vi "EMC_REL_Move.vi"(8 "error in (no error)":errorcluster, 10 "Motion Parameters":T1={"position"=1000.0, "velocity"=1000.0, "acceleration"=10000.0, "deceleration"=10000.0, "accel. jerk"=10000.0, "decel. jerk"=10000.0}, 11 "axis":refnum<k21>) -> (0 "error out":errorcluster)   [LabVIEW 2015]
uses:
  EMC_Typedef_Motor_Parameters.ctl
  <vilib>/Motion/PropertyNodes/nimc.createStraightLineMoveInstance.axis.vi
  <vilib>/Motion/PropertyNodes/nimc.destroyInterfaceInstance.vi
  <resource>/objmgr/nimotion.rc
panel:
  out "Numeric":i32
  in  "table":refnum<k21>
  in  "coordinate":refnum<k21>
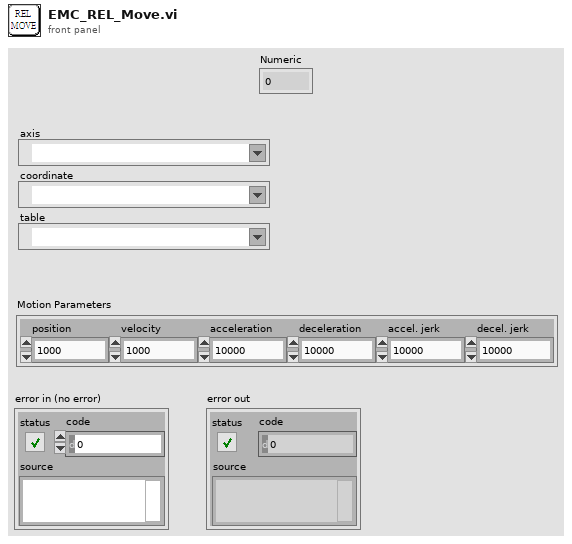
[diagram p1: front panel]
types:
  T1 = typedef "EMC_Typedef_Motor_Parameters.ctl" = cluster{"position":dbl, "velocity":dbl, "acceleration":dbl, "deceleration":dbl, "accel. jerk":dbl, "decel. jerk":dbl}
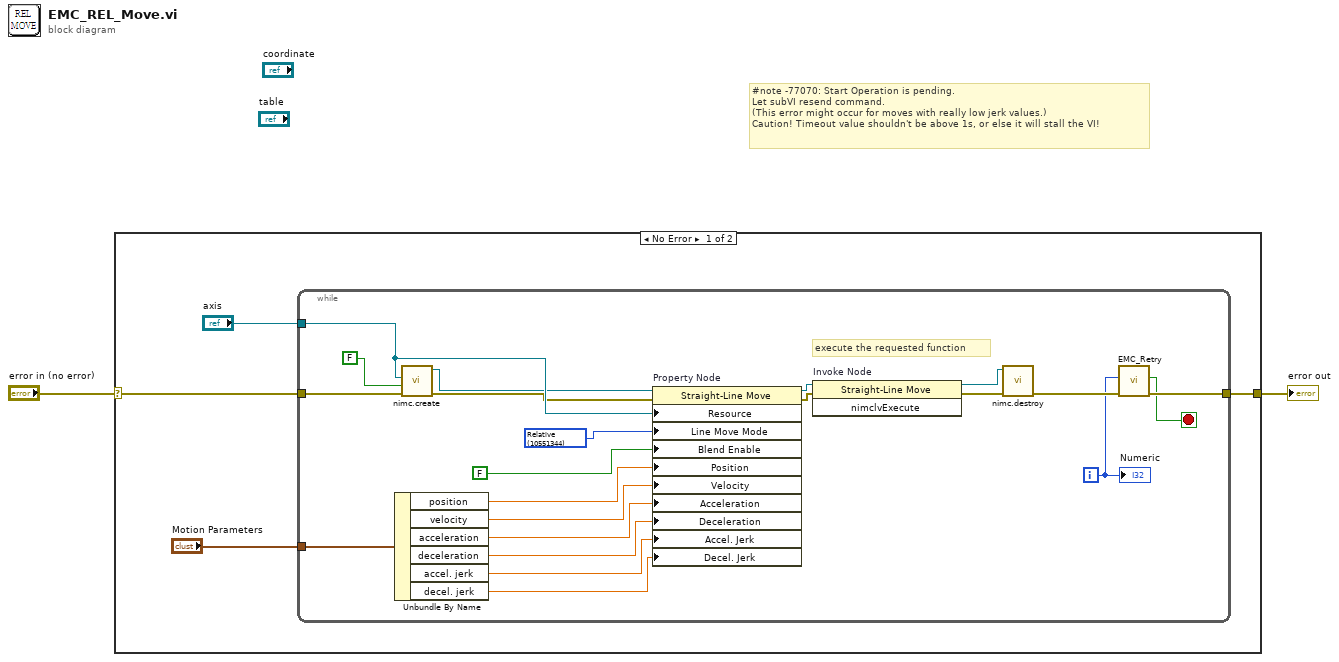
[diagram p0: block diagram]
diagram:
  # "#note -77070: Start Operation is pending.\nLet subVI resend command.\n(This error might occur for moves with really low jerk values.)\nCaution! Timeout value shouldn't be above 1s, or else it will stall the VI!"
  n1 = case shown="No Error" "error in (no error)" {
    selector: "error in (no error)" -> [w6 w29]
    tunnel: [w3 w29] -> w2
    frame No Error {
      n2 = while {
        tunnel: w6 -> [w28]
        tunnel: "axis" -> [w27]
        tunnel: "Motion Parameters" -> [w26]
        tunnel: [w9] -> w3
        i -> [w7]
        stop <- w8 stop-if-true
        w13 = 10551344 items=["Relative"=10551344, "Absolute"=10551337, "Relative To Capture"=10551345, "Velocity"=10551346, "Polyline"=11600101] ("line move mode")
        # "execute the requested function"
        n3 = Unbundle By Name(w26) -> ("position"=w19:dbl, "velocity"=w18:dbl, "acceleration"=w17:dbl, "deceleration"=w16:dbl, "accel. jerk"=w15:dbl, "decel. jerk"=w14:dbl)
        n4 = call-poly <vilib>:"nimc.create.vi"("error in"=w28, "async?"=FALSE ("execute asynchronously?"), "axis"=w27) -> ("error out"=w11:errorcluster, "line"=w12:refnum<k20>)  [unwired: 6 in, 1 out]
        n5 = property on="Property Node" class="Straight-Line Move"(reference=w12, error in=w11, "Resource"=w27, "Line Move Mode"=w13, "Blend Enable"=FALSE ("blend enable"), "Position"=w19, "Velocity"=w18, "Acceleration"=w17, "Deceleration"=w16, "Accel. Jerk"=w15, "Decel. Jerk"=w14) -> (reference out=w25:refnum<k20>, error out=w24:errorcluster)
        n6 = invoke on="Invoke Node" class="Straight-Line Move" method="nimclvExecute"(reference=w25, error in=w24) -> (reference out=w22:refnum<k20>, error out=w21:errorcluster)  [unwired: 1 in, 1 out]
        n7 = call-poly <vilib>:"nimc.destroy.vi"("error in"=w21, "motion handle"=w22) -> ("error out"=w10:errorcluster)  [unwired: 9 in]
        n8 = call "EMC_Retry.vi"("error in (no error)"=w10, "Count in"=w7) -> ("error out"=w9:errorcluster, "Exit"=w8:bool)  [unwired: 8 in]
        "Numeric" <- w7
      }
    }
    frame Error {
    }
  }
  "error out" <- w2
